vi "wheels.vi"(1 "Enum":enum16{"Low", "Medium", "High"}(ring)) -> (0 "Aim":dbl)   [LabVIEW 2012]
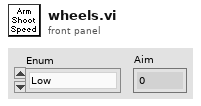
[diagram p1: front panel]
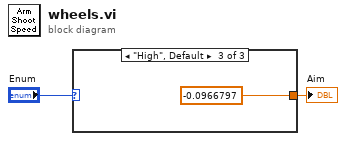
[diagram p0: block diagram]
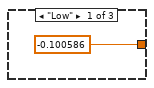
[diagram p2: hidden frame]
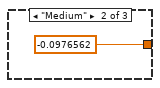
[diagram p3: hidden frame]
diagram:
  n1 = case shown="\"High\", Default" "Enum" {
    tunnel: [-0.100586 -0.0976562 -0.0966797] -> w1
    frame "Low" {
    }
    frame "Medium" {
    }
    frame "High", Default {
    }
  }
  "Aim" <- w1
